vi "Lakeshore 336 Apply Channel Settings.vi"(8 "error in (no error)":errorcluster, 9 "Manual Settings":T1={"Input (0:None)"=0, "Power Up Enable (F: Off)"=FALSE, "Mode (0:Off)"=0, "Max Current (0:User Specified)"=0, "Heater Out Display (1:Current)"=1, "Max User Current (2.000)"=2.0, "Heater Resistance (1:25 Ohms)"=1, "PID"={"P"=0.0, "I"=0.0, "D"=0.0}, "Name"=""} {"Heater Resistance (1:25 Ohms)" items=["25 Ohms"=1, "50 Ohms"=2]; "Max User Current (2.000)" format="%.3f"; "Heater Out Display (1:Current)" items=["Current"=1, "Power"=2]; "Max Current (0:User Specified)" items=["User Specified", "0.707 A", "1.0 A", "1.141 A", "2.0 A"]; "Mode (0:Off)" items=["Off", "Closed Loop PID", "Zone", "Open Loop"]; "Input (0:None)" items=["None", "A", "B", "C", "D"]}, 10 "Channel (1)":i32=1 min=1 max=4 step=1, 11 "Addr":refnum<visa-resource-name>) -> (0 "error out":errorcluster, 2 "Channel dup":i32=1 min=1 max=4 step=1, 3 "Addr dup":refnum<visa-resource-name>)   [LabVIEW 2022 SP3, in "Lakeshore 336.lvclass"]
uses:
  Lakeshore 336.lvclass
  Lakeshore 336 Channel Settings cluster.ctl
  Lakeshore 336 PID cluster.ctl
  Lakeshore 336.lvclass/Lakeshore 336.ctl
  <instrlib>/Lake Shore 336/Lake Shore 336.lvlib
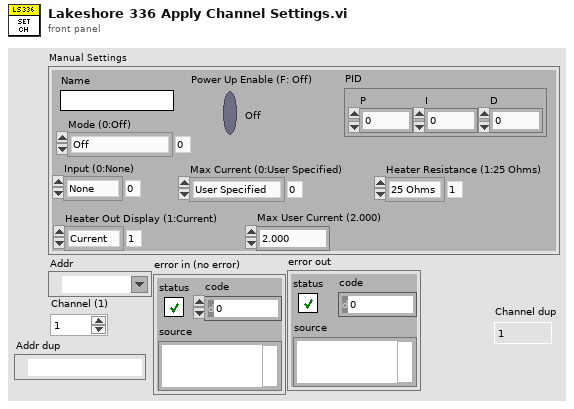
[diagram p1: front panel]
types:
  T1 = typedef "Lakeshore 336.lvclass/Lakeshore 336 Channel Settings cluster.ctl" = cluster{"Input (0:None)":u16, "Power Up Enable (F: Off)":bool, "Mode (0:Off)":u16, "Max Current (0:User Specified)":u16, "Heater Out Display (1:Current)":u16, "Max User Current (2.000)":dbl, "Heater Resistance (1:25 Ohms)":u16, "PID":T2, "Name":string}
  T2 = typedef "Lakeshore 336.lvclass/Lakeshore 336 PID cluster.ctl" = cluster{"P":dbl, "I":dbl, "D":dbl}
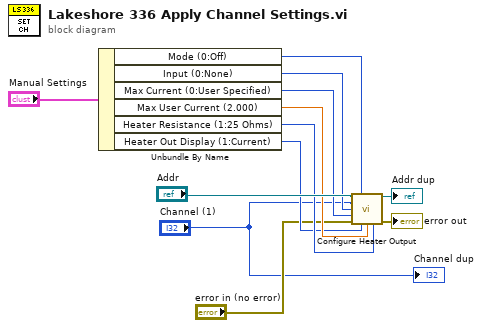
[diagram p0: block diagram]
diagram:
  n1 = Unbundle By Name("Manual Settings") -> ("Mode (0:Off)"=w10:u16, "Input (0:None)"=w9:u16, "Max Current (0:User Specified)"=w8:u16, "Max User Current (2.000)"=w7:dbl, "Heater Resistance (1:25 Ohms)"=w6:u16, "Heater Out Display (1:Current)"=w5:u16)
  n2 = call <instrlib>:"Configure Heater Output.vi"("VISA resource name"="Addr", "Mode (0:Off)"=w10, "Heater Output (1:1)"="Channel (1)", "Input (0:None)"=w9, "Max Current (0:User Specified)"=w8, "error in (no error)"="error in (no error)", "Heater Out Display (1:Current)"=w5, "Max User Current (2.000)"=w7, "Heater Resistance (1:25 Ohms)"=w6) -> ("VISA resource name out"=→"Addr dup":refnum<visa-resource-name>, "error out"=→"error out":errorcluster)  [unwired: 5 in]
  "Channel dup" <- "Channel (1)"
